vi "ToF to Distance.vi"(1 "Time of Flight":dbl) -> (0 "Distance":dbl)   [LabVIEW 2015, in "SonarSensor.lvclass"]
uses:
  SonarSensor.lvclass
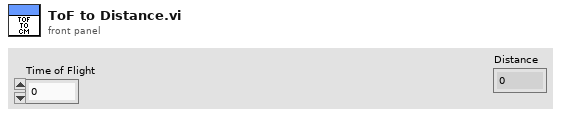
[diagram p1: front panel]
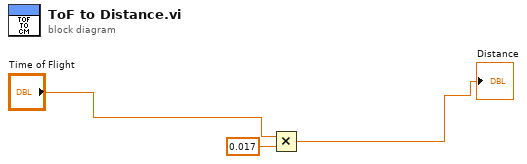
[diagram p0: block diagram]
diagram:
  n1 = Multiply(x="Time of Flight", y=0.017) -> (x*y=→"Distance":dbl)
